vi "Find unique elements.vi"(11 "Numeric":u32) -> (3 "Array":u32[](array[numeric]))   [LabVIEW 2015]
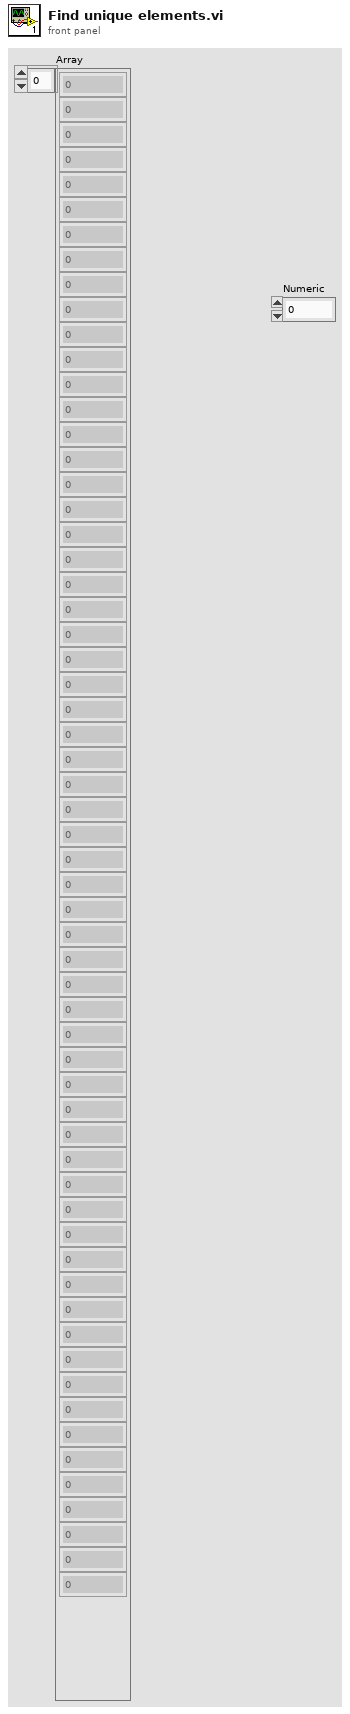
[diagram p1: front panel]
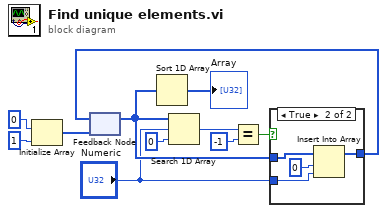
[diagram p0: block diagram]
diagram:
  n1 = Initialize Array(u32 0, 1) -> (w2:u32[])
  n2 = feedback #1(w2) -> (w10:u32[])
  n3 = Sort 1D Array(array=w10) -> (sorted array=→"Array":u32[])
  n4 = Search 1D Array(1D array=w10, element="Numeric", start index (0)=u32 0) -> (index of element=w6:i32)
  n5 = Equal?(x=w6, y=-1) -> (x = y?=w8:bool)
  n6 = case shown="True" w8 {
    tunnel: "Numeric" -> [_ w16]
    tunnel: [w12 w15] -> w5
    tunnel: w10 -> [w12 w14]
    frame False {
    }
    frame True {
      n7 = Insert Into Array(array=w14, index=u32 0, new element=w16) -> (w15:u32[])
    }
  }
  n8 = feedback-in #1(w5) -> ()
